vi "sub_file_log_1.vi"(0 "LOG PATH IN":path, 1 "TIMESTAMP (MMM DD, YY | hh:mm:ss,sss)":string, 2 "UID":string, 3 "ACTIVITY":string, 5 "ERROR IN":errorcluster) -> (14 "LOG PATH OUT":path, 19 "ERROR OUT":errorcluster)   [LabVIEW 2018]
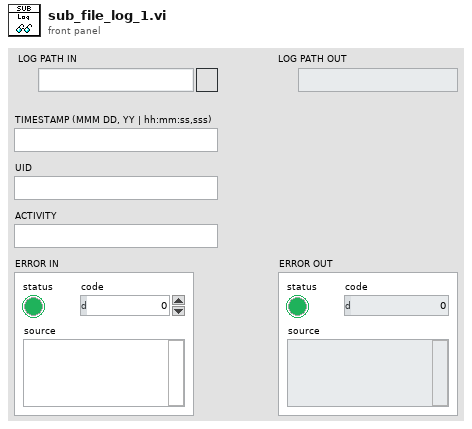
[diagram p1: front panel]
types:
  T1 = enum16{"open", "replace", "create", "open or create", "replace or create", "replace or create with confirmation"}
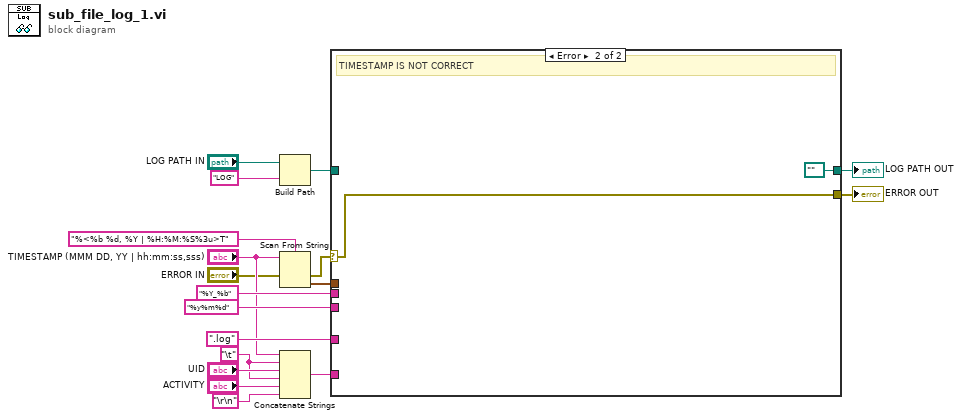
[diagram p0: block diagram]
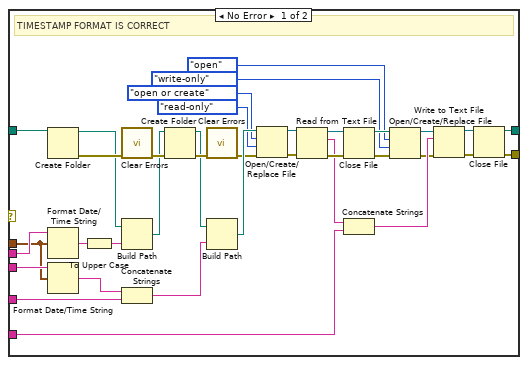
[diagram p2: hidden frame]
diagram:
  w17 = "\t"
  n1 = Build Path(base path="LOG PATH IN", name or relative path="LOG" ("string")) -> (appended path=w13:path)
  n2 = Scan From String(format string="%<%b %d, %Y | %H:%M:%S%3u>T", input string="TIMESTAMP (MMM DD, YY | hh:mm:ss,sss)", error in="ERROR IN") -> (error out=w2:errorcluster, output 1=w8:timestamp)  [unwired: 2 in, 2 out]
  n3 = Concatenate Strings("TIMESTAMP (MMM DD, YY | hh:mm:ss,sss)", w17, "UID", w17, "ACTIVITY", "\r\n") -> (w4:string)
  n4 = case shown="Error" w2 {
    selector: w2 -> [_ w56]
    tunnel: w13 -> [w54 _]
    tunnel: ".log" ("string") -> [w47 _]
    tunnel: "%Y_%b" ("time format string (%c)") -> [w43 _]
    tunnel: "%y%m%d" ("time format string (%c)") -> [w42 _]
    tunnel: w8 -> [w41 _]
    tunnel: [w35 w56] -> w6
    tunnel: w4 -> [w29 _]
    tunnel: [w19 path "" ("path")] -> w1
    frame No Error {
      # "TIMESTAMP FORMAT IS CORRECT"
      n5 = Create Folder(path (use dialog)=w54) -> (created path=w51:path, error out=w53:errorcluster)  [unwired: 2 in, 1 out]
      n6 = Format Date/Time String(time format string (%c)=w43, seconds (now)=w41) -> (date/time string=w38:string)  [unwired: 1 in]
      n7 = Format Date/Time String(time format string (%c)=w42, seconds (now)=w41) -> (date/time string=w40:string)  [unwired: 1 in]
      n8 = To Upper Case(1:w38) -> (0:w39:string)
      n9 = call <vilib>:"Clear Errors.vi"("error in (no error)"=w53) -> ("error out"=w52:errorcluster)  [unwired: 5 in, 1 out]
      n10 = Build Path(base path=w51, name or relative path=w39) -> (appended path=w50:path)
      n11 = Concatenate Strings(w40, w47) -> (w46:string)
      n12 = Create Folder(path (use dialog)=w50, error in=w52) -> (created path=w48:path, error out=w49:errorcluster)  [unwired: 1 in, 1 out]
      n13 = call <vilib>:"Clear Errors.vi"("error in (no error)"=w49) -> ("error out"=w44:errorcluster)  [unwired: 5 in, 1 out]
      n14 = Build Path(base path=w48, name or relative path=w46) -> (appended path=w45:path)
      n15 = Open/Create/Replace File(file path (use dialog)=w45, error in=w44, operation (0:open)=T1."open or create", access (0:read/write)=enum16{"read/write", "read-only", "write-only"}."read-only") -> (refnum out=w33:refnum<file>, error out=w34:errorcluster)  [unwired: 2 in, 1 out]
      n16 = Read from Text File(file (use dialog)=w33, error in=w34) -> (refnum out=w31:refnum<file>, text=w30:string, error out=w32:errorcluster)  [unwired: 2 in, 1 out]
      n17 = Close File(refnum=w31, error in=w32) -> (path=w27:path, error out=w28:errorcluster)
      n18 = Concatenate Strings(w30, w29) -> (w26:string)
      n19 = Open/Create/Replace File(file path (use dialog)=w27, error in=w28, operation (0:open)=T1."open", access (0:read/write)=enum16{"read/write", "read-only", "write-only"}."write-only") -> (refnum out=w24:refnum<file>, error out=w25:errorcluster)  [unwired: 2 in, 1 out]
      n20 = Write to Text File(file (use dialog)=w24, text=w26, error in=w25) -> (refnum out=w36:refnum<file>, error out=w37:errorcluster)  [unwired: 1 in, 1 out]
      n21 = Close File(refnum=w36, error in=w37) -> (path=w19:path, error out=w35:errorcluster)
    }
    frame Error {
      # "TIMESTAMP IS NOT CORRECT"
    }
  }
  "ERROR OUT" <- w6
  "LOG PATH OUT" <- w1
